vi "Global.vi"() -> ()   [LabVIEW 2013]
panel:
  in  "GStop":bool
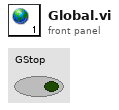
[diagram p1: front panel]
diagram:
